vi "TurnMath.vi"(10 "Yaw in":dbl, 11 "Target Yaw in":dbl) -> (2 "Yaw out":dbl, 3 "Target Yaw out":dbl)   [LabVIEW 2017]
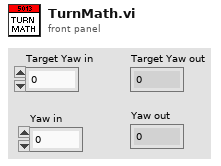
[diagram p1: front panel]
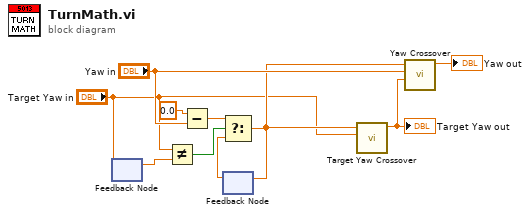
[diagram p0: block diagram]
diagram:
  n1 = feedback #1() -> (w8:dbl)  [unwired: 1 in]
  n2 = feedback-in #1("Target Yaw in") -> ()
  n3 = Not Equal?(x="Target Yaw in", y=w8) -> (x != y?=w7:bool)
  n4 = Subtract(x=0.0 ("Y-Axis"), y="Yaw in") -> (x-y=w10:dbl)
  n5 = feedback #2() -> (w6:dbl)  [unwired: 1 in]
  n6 = Select(t=w10, s=w7, f=w6) -> (s? t:f=w3:dbl)
  n7 = feedback-in #2(w3) -> ()
  n8 = call "Target Yaw Crossover.vi"("Yaw in"="Target Yaw in", "Adjustment"=w3) -> ("Numeric out"=w1:dbl)  [unwired: 9 in]
  "Target Yaw out" <- w1
  n9 = call "Yaw Crossover.vi"("Target Adjusted Yaw"=w1, "Yaw in"="Yaw in", "Adjustment"=w3) -> ("Numeric out"=→"Yaw out":dbl)  [unwired: 8 in]
